vi "GenericConfigureDrive.vi"(0 "Address":u8, 1 "Port Name":string, 2 "Static Drive Configuration":T1={"Correction Gain % (CG)"=1, "Dead Band (DB)"=10, "Dead Band Window (DW)"=10, "Encoder Resolution (ER)"=4000, "Step Mode  (FSB)"=0, "Position Maintenance (FSC)"=0, "Stop on Stall (FSD)"=0, "Activate OP1 on stall (FSE)"=0, "Stop on Trigger 3 (FSF)"=0, "OP2 in Deadband (FSG)"=0, "Stall Detect (FSH)"=0, "Limit Disable (LD)"=0, "Motor Resolution (MR)"=enum."20000", "Limit Switch Sense (OSA)"=0, "Home Position (OSB)"=1, "Home Switch Sense (OSC)"=0, "Encoder Z for Home (OSD)"=0, "Reference edge of Home (OSH)"=0, "RS232 Echo Control (SSA)"=0, "Buffer at Limit (SSG)"=1, "Buffer at Stop (SSH)"=1, "Indexer Mode  (FSA)"=1, "Type"="", "ConfigString"="", "De Power Motor"=enum."FALSE"} {"Indexer Mode  (FSA)" items=["Incremental", "Absolute"]; "Buffer at Stop (SSH)" items=["Clear buffer", "Save and Continue"]; "Buffer at Limit (SSG)" items=["Clear buffer", "Save and Continue"]; "RS232 Echo Control (SSA)" items=["Echo ON", "Echo OFF"]; "Reference edge of Home (OSH)" items=["CW", "CCW"]; "Encoder Z for Home (OSD)" items=["Don't use", "Enable"]; "Home Switch Sense (OSC)" items=["Normally Open", "Normally Closed"]; "Home Position (OSB)" items=["Anywhere in Switch", "Edge of Switch"]; "Limit Switch Sense (OSA)" items=["Normally Closed", "Normally Open"]; "Limit Disable (LD)" items=["Both Enabled", "CW Disabled", "CCW Disabled", "Both Disabled"]; "Stall Detect (FSH)" items=["Disable", "Enable"]; "OP2 in Deadband (FSG)" items=["Don't Use", "ACTIVATE"]; "Stop on Trigger 3 (FSF)" items=["Ignore", "STOP!"]; "Activate OP1 on stall (FSE)" items=["Do not Activate", "ACTIVATE!"]; "Stop on Stall (FSD)" items=["Continue", "STOP"]; "Position Maintenance (FSC)" items=["Disabled", "Enabled"]; "Step Mode  (FSB)" items=["Motor", "Encoder"]; "Encoder Resolution (ER)" min=1 max=50000; "Dead Band Window (DW)" min=0 max=999999999; "Dead Band (DB)" min=0 max=999999999; "Correction Gain % (CG)" items=["n/a", "12.5", "25", "37.5", "50", "62.5", "75", "87.5", "100"]}, 3 "Channel Name":string) -> (8 "Good Echo":bool)   [LabVIEW 2015]
uses:
  ~subVIs/DriveStaticConfig.ctl
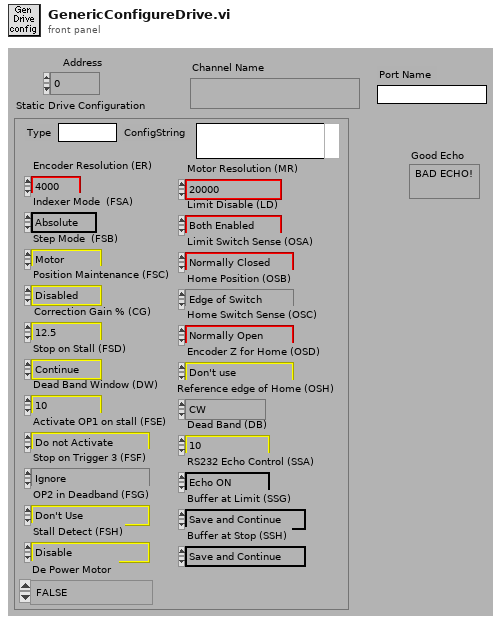
[diagram p1: front panel]
types:
  T1 = typedef "DriveStaticConfig.ctl" = cluster{"Correction Gain % (CG)":u16, "Dead Band (DB)":i32, "Dead Band Window (DW)":i32, "Encoder Resolution (ER)":i32, "Step Mode  (FSB)":u16, "Position Maintenance (FSC)":u16, "Stop on Stall (FSD)":u16, "Activate OP1 on stall (FSE)":u16, "Stop on Trigger 3 (FSF)":u16, "OP2 in Deadband (FSG)":u16, "Stall Detect (FSH)":u16, "Limit Disable (LD)":u16, "Motor Resolution (MR)":enum16{"200", "400", "1000", "2000", "4000", "5000", "10000", "12800", "18000", "20000", "21600", "25000", "25400", "25600", "36000", "50000", "278528", "425984", "507904", "614400", "655360", "819200", "1024000"}, "Limit Switch Sense (OSA)":u16, "Home Position (OSB)":u16, "Home Switch Sense (OSC)":u16, "Encoder Z for Home (OSD)":u16, "Reference edge of Home (OSH)":u16, "RS232 Echo Control (SSA)":u16, "Buffer at Limit (SSG)":u16, "Buffer at Stop (SSH)":u16, "Indexer Mode  (FSA)":u16, "Type":string, "ConfigString":string, "De Power Motor":enum16{"TRUE", "FALSE"}}
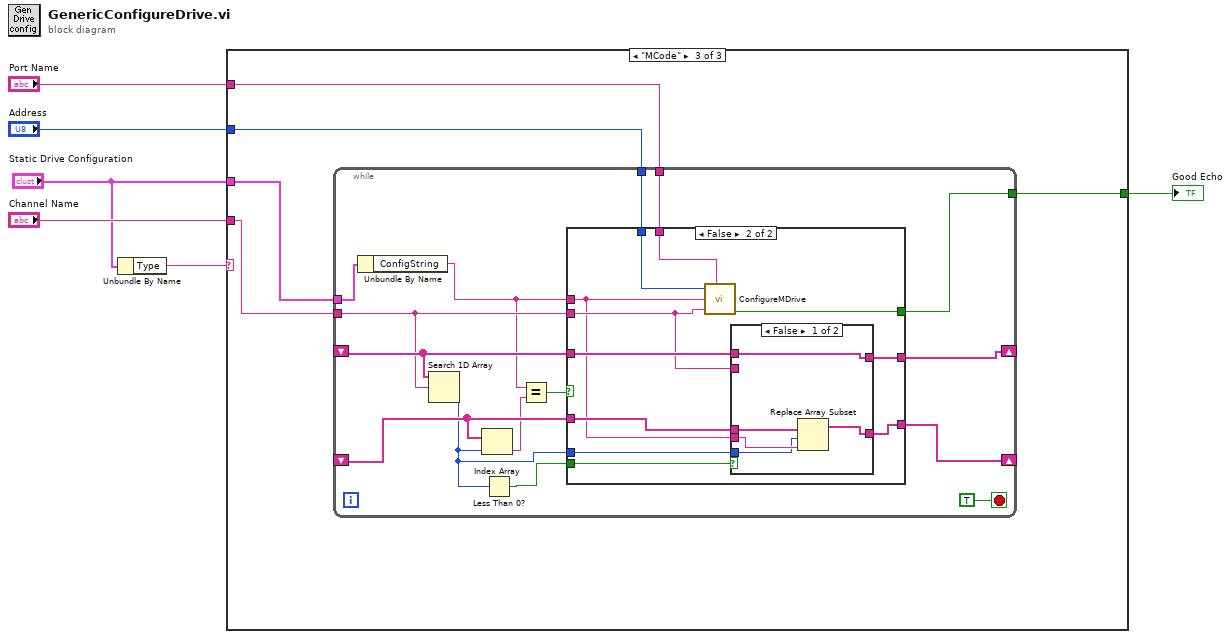
[diagram p0: block diagram]
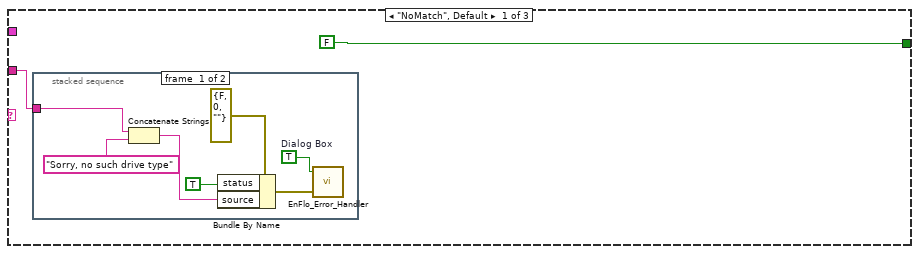
[diagram p2: hidden frame]
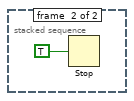
[diagram p3: hidden frame]
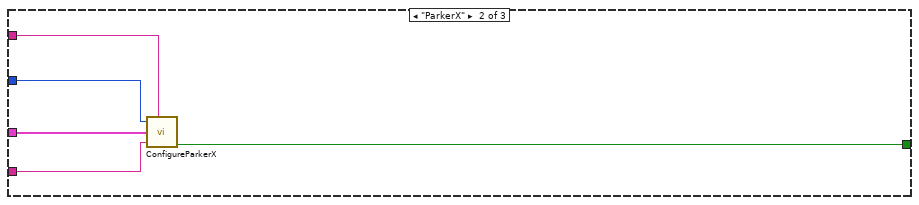
[diagram p4: hidden frame]
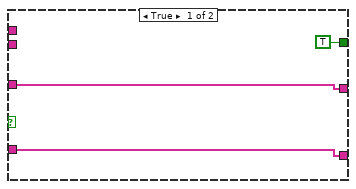
[diagram p5: hidden frame]
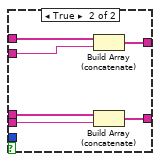
[diagram p6: hidden frame]
diagram:
  n1 = Unbundle By Name("Static Drive Configuration") -> ("Type"=w2:string)
  n2 = case shown="\"MCode\"" w2 {
    tunnel: "Address" -> [_ w21 w26]
    tunnel: "Static Drive Configuration" -> [_ w20 w22]
    tunnel: "Port Name" -> [_ w19 w25]
    tunnel: "Channel Name" -> [w7 w18 w24]
    tunnel: [FALSE ("Good Echo") w17 w23] -> w3
    frame "NoMatch", Default {
      n3 = stacked-sequence {
        tunnel: w7 -> [w9 _]
        frame #0 {
          w10 = TRUE  # Dialog Box
          n4 = Concatenate Strings(w9, "Sorry, no such drive type") -> (w11:string)
          n5 = Bundle By Name(cluster=errorcluster {"status"=FALSE, "code"=0, "source"=""} ("error in (no error)"), "status"=TRUE ("Bundle Element"), "source"=w11) -> (w14:errorcluster)
          n6 = call "EnFlo_Error_Handler.vi"("error in (no error)"=w14, "Dialog Box (T)"=w10) -> ()  [unwired: 1 in, 3 out]
        }
        frame #1 {
          n7 = Stop(stop? (T)=TRUE) -> ()
        }
      }
    }
    frame "ParkerX" {
      n8 = call "ConfigureParkerX.vi"("Address"=w21, "Port Name"=w19, "Static Drive Configuration"=w20, "Channel Name"=w18) -> ("Good Echo"=w17:bool)  [unwired: 4 out]
    }
    frame "MCode" {
      n9 = while {
        tunnel: w26 -> [w41]
        tunnel: w25 -> [w40]
        tunnel: w24 -> [w34]
        tunnel: [w39] -> w23
        tunnel: w22 -> [w28]
        shift-right: [w38] -> _
        shift-left: _ -> [w33]
        shift-right: [w36] -> _
        shift-left: _ -> [w35]
        stop <- TRUE stop-if-true
        n10 = Unbundle By Name(w28) -> ("ConfigString"=w27:string)
        n11 = Search 1D Array(1D array=w35, element=w34) -> (index of element=w29:i32)  [unwired: 1 in]
        n12 = Index Array(array=w33, index=w29) -> (element=w32:string)
        n13 = Less Than 0?(x=w29) -> (x < 0?=w30:bool)
        n14 = Equal?(x=w27, y=w32) -> (x = y?=w31:bool)
        n15 = case shown="False" w31 {
          tunnel: w41 -> [_ w55]
          tunnel: w40 -> [_ w54]
          tunnel: w34 -> [_ w48]
          tunnel: [TRUE ("Good Echo") w53] -> w39
          tunnel: w27 -> [_ w45]
          tunnel: [w43 w52] -> w38
          tunnel: w33 -> [w43 w51]
          tunnel: w35 -> [w42 w50]
          tunnel: [w42 w49] -> w36
          tunnel: w30 -> [_ w47]
          tunnel: w29 -> [_ w46]
          frame True {
          }
          frame False {
            n16 = call "ConfigureMDrive.vi"("Address"=w55, "Port Name"=w54, "ConfigString"=w45, "Channel Name"=w48) -> ("Good Echo"=w53:bool)  [unwired: 4 out]
            n17 = case shown="False" w47 {
              tunnel: [w56 w66] -> w52
              tunnel: w51 -> [w60 w65]
              tunnel: w50 -> [w57 w64]
              tunnel: [w57 w63] -> w49
              tunnel: w45 -> [w59 w62]
              tunnel: w48 -> [_ w61]
              tunnel: w46 -> [w58 _]
              frame False {
                n18 = Replace Array Subset(array=w60, new element=w59, index=w58) -> (w56:string[])
              }
              frame True {
                n19 = Build Array (concatenate)(w64, w61) -> (w63:string[])
                n20 = Build Array (concatenate)(w65, w62) -> (w66:string[])
              }
            }
          }
        }
      }
    }
  }
  "Good Echo" <- w3
